vi "Actor Core.vi"(8 "error in":errorcluster caption="错误输入", 11 "DAQ in":refnum<class "DAQ.lvclass"> caption="操作者输入") -> (0 "error out":errorcluster caption="错误输出", 3 "Actor out":refnum<class "Actor.lvclass"> caption="操作者输出")   [LabVIEW 2017, in "DAQ.lvlib" / "DAQ.lvclass"]
doc: "(<B>Filename</B>: Actor Framework.lvlib:Actor.lvclass:Actor Core.vi)\n\nReceives messages to the actor, reacts to them, and initiates any error handling that may shut the actor down.\n\nDescendant classes may override this VI to append parallel tasks for the actor to complete while it handles messages.使用调用父方法节点实现重写。"
uses:
  DAQ.lvclass
  E:/Program Files (x86)/National Instruments/LabVIEW 2017/vi.lib/ActorFramework/Actor/Actor.lvclass
  <vilib>/ActorFramework/Actor/Actor.lvclass
  <vilib>/ActorFramework/Actor/Actor.lvclass/Actor.ctl
  DAQ.lvclass/DAQ.ctl
  <vilib>/ActorFramework/Message Enqueuer/Message Enqueuer.lvclass/Message Enqueuer.ctl
  <vilib>/ActorFramework/Message Enqueuer/Enqueue.vi
  E:/Program Files (x86)/National Instruments/LabVIEW 2017/vi.lib/ActorFramework/Message/Message.lvclass
  <vilib>/ActorFramework/Stop Msg/Stop Msg.lvclass
  <vilib>/ActorFramework/Message Priority Queue/Priority Enqueue.vi
panel:
  in  "停止":bool
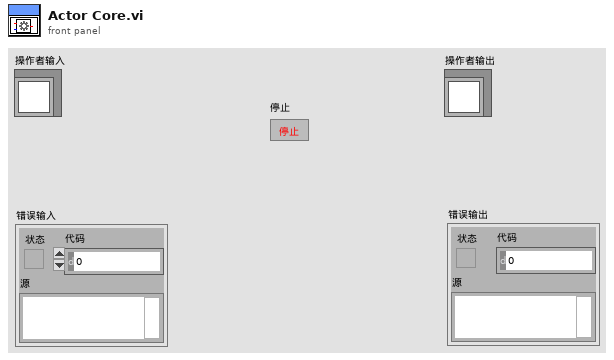
[diagram p1: front panel]
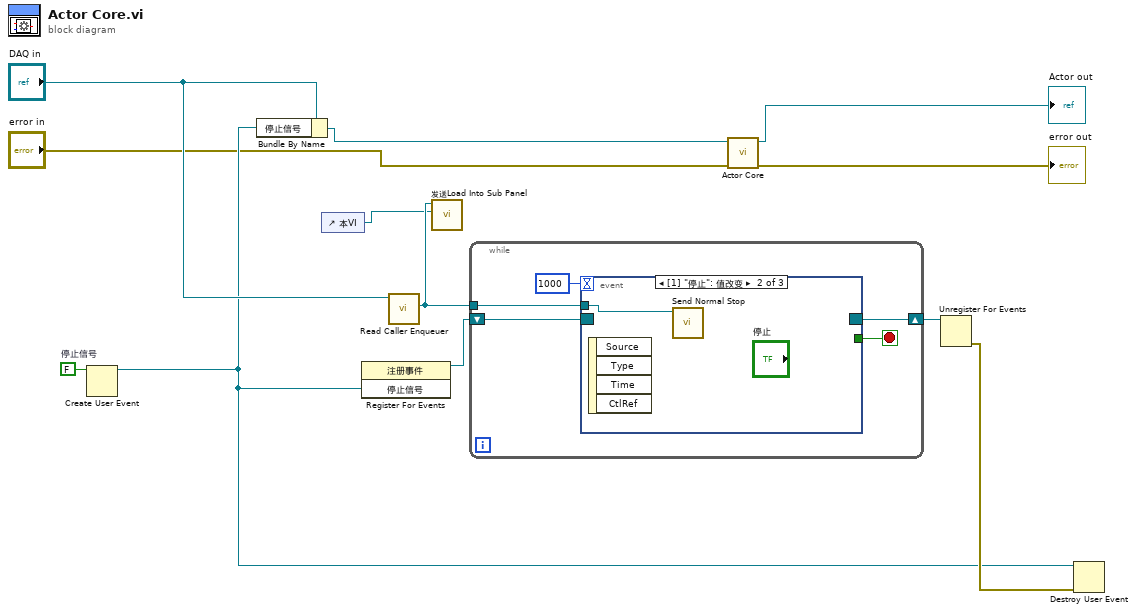
[diagram p0: block diagram]
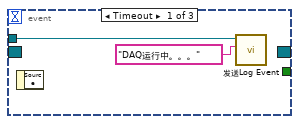
[diagram p2: hidden frame]
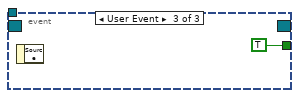
[diagram p3: hidden frame]
diagram:
  w11 = FALSE  # 停止信号
  n1 = Create User Event ("创建用户事件")(user event datatype=w11) -> (user event=w6:refnum<user-event>)  [unwired: 1 in, 1 out]
  n2 = Bundle By Name(cluster="DAQ in", "停止信号"=w6) -> (w9:refnum<class "DAQ.lvclass">)
  n3 = control-ref of="本VI"() -> (w1:refnum<vi>)
  n4 = register-events(w6) -> (reference out=w8:refnum<event-registration>)  [unwired: 2 in, 1 out]
  n5 = call <vilib>:"Read Caller Enqueuer.vi"("Actor"="DAQ in") -> ("Caller Enqueuer"=w2:refnum<class "Message Enqueuer.lvclass">)  [unwired: 10 in]
  n6 = call "发送Load Into Sub Panel.vi"("VI引用"=w1, "Message Enqueuer"=w2) -> ()  [unwired: 8 in, 2 out]
  n7 = while {
    tunnel: w2 -> [w17]
    shift-right: [w13] -> w5
    shift-left: w8 -> [w15]
    stop <- w14 stop-if-true
    n8 = event shown="[1] \"停止\": 值改变" {
      selector: w15 -> [_ _ _]
      dyn-events: [_ _ _] -> w13
      timeout: 1000 -> [_ _ _]
      tunnel: w17 -> [w19 w20 _]
      tunnel: [_ _ TRUE] -> w14
      event Timeout {
        n9 = event-data() -> ()  [unwired: 1 in, 1 out]
        n10 = call "发送Log Event.vi"("事件文本"="DAQ运行中。。。", "Message Enqueuer"=w19) -> ()  [unwired: 8 in, 2 out]
      }
      event "停止": Value Change {
        n11 = event-data() -> ()  [unwired: 1 in, 4 out]
        n12 = call <vilib>:"Send Normal Stop.vi"("Message Enqueuer"=w20) -> ()  [unwired: 10 in, 1 out]
      }
      event User Event {
        n13 = event-data() -> ()  [unwired: 1 in, 1 out]
      }
    }
  }
  n14 = call-parent "Actor Core.vi"("error in"="error in", "Actor in"=w9) -> ("error out"=→"error out":errorcluster, "Actor out"=→"Actor out":refnum<class "Actor.lvclass">)  [unwired: 8 in]
  n15 = Unregister For Events(event registration refnum=w5) -> (error out=w7:errorcluster)  [unwired: 1 in]
  n16 = Destroy User Event(user event=w6, error in=w7) -> ()  [unwired: 1 out]
